vi "testNotARefnum.vi"() -> ()   [LabVIEW 2017, in "Assertion.Tests.lvlib" / "AssertRefnum.lvlib"]
uses:
  AssertRefnum.lvlib
  Assertion/Assertion.lvlib
panel:
  out "error out":errorcluster
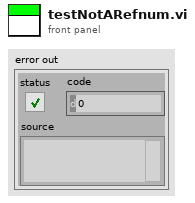
[diagram p1: front panel]
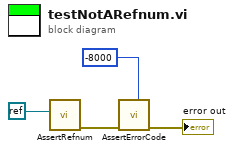
[diagram p0: block diagram]
diagram:
  n1 = call "AssertRefnum.vi"("Refnum"=refnum<k0> refnum) -> ("error out"=w3:errorcluster)  [unwired: 10 in]
  n2 = call "AssertErrorCode.vi"("Expected"=-8000, "error in (no error)"=w3) -> ("error out"=→"error out":errorcluster)  [unwired: 9 in]
